vi "Single HWSync LITE.vi"() -> ()   [LabVIEW 2014]
doc: "Use this template to build a producer/consumer design pattern with events to produce queue items. Use this design pattern instead of the User Interface Event Handler pattern for user interfaces when you want to execute code asynchronously in response to an event without slowing the user interface responsiveness."
uses:
  TypeDefs/HAL Config Data.ctl
  APIs/Data Queue/Acquisition Data 1 Sample Cluster.ctl
  APIs/Data Queue/Control Data Cluster.ctl
  APIs/Message Queue/Enqueue Message (Array).vi
  APIs/Message Queue/WINFAS 2 Message Queue.lvlib
  HWSyncLoop/HWSyncLoop.lvlib
  APIs/Data Queue/WINFAS 2 Data Queue.lvlib
panel:
  in  "Config":bool
  in  "LOAD DRIVER":bool
  in  "Disconnect":bool
  in  "Connect":bool
  in  "Sequence:Stop":bool
  in  "Sequence:Start":bool
  in  "Auto-Refresh:Stop":bool
  in  "Auto-Refresh:Start":bool
  in  "Stop Cycle":bool
  in  "Stop Measurement":bool
  in  "Start Measurement":bool
  in  "Start Cycle":bool
  out "TDX":sgl[][](graph)
  out "Valores TDX":sgl[](array[numeric]) format="%0+10.6fmm"
  out "TDX N°":i32[](array[numeric])
  in  "Encoder Zero":bool
  out "DO":bool[][](array[boolean])
  out "DI":bool[][](array[boolean])
  in  "DO Button":bool[][](array[boolean])=[[FALSE, FALSE, FALSE, FALSE, FALSE, FALSE, FALSE, FALSE], [FALSE, FALSE, FALSE, FALSE, FALSE, FALSE, FALSE, FALSE]]
  out "Encoder":sgl(knob) scale=-360.0..360.0 scale format="%.0f°"
  out "Errores":string
  out "Status Bar":string="LOAD"
  out "Driver:":string
  # "Single HWSync LITE"
  # "Entradas Digitales (0-15)"
  # "Salidas Digitales (0-15)"
  # "Salidas Digitales (0-15)"
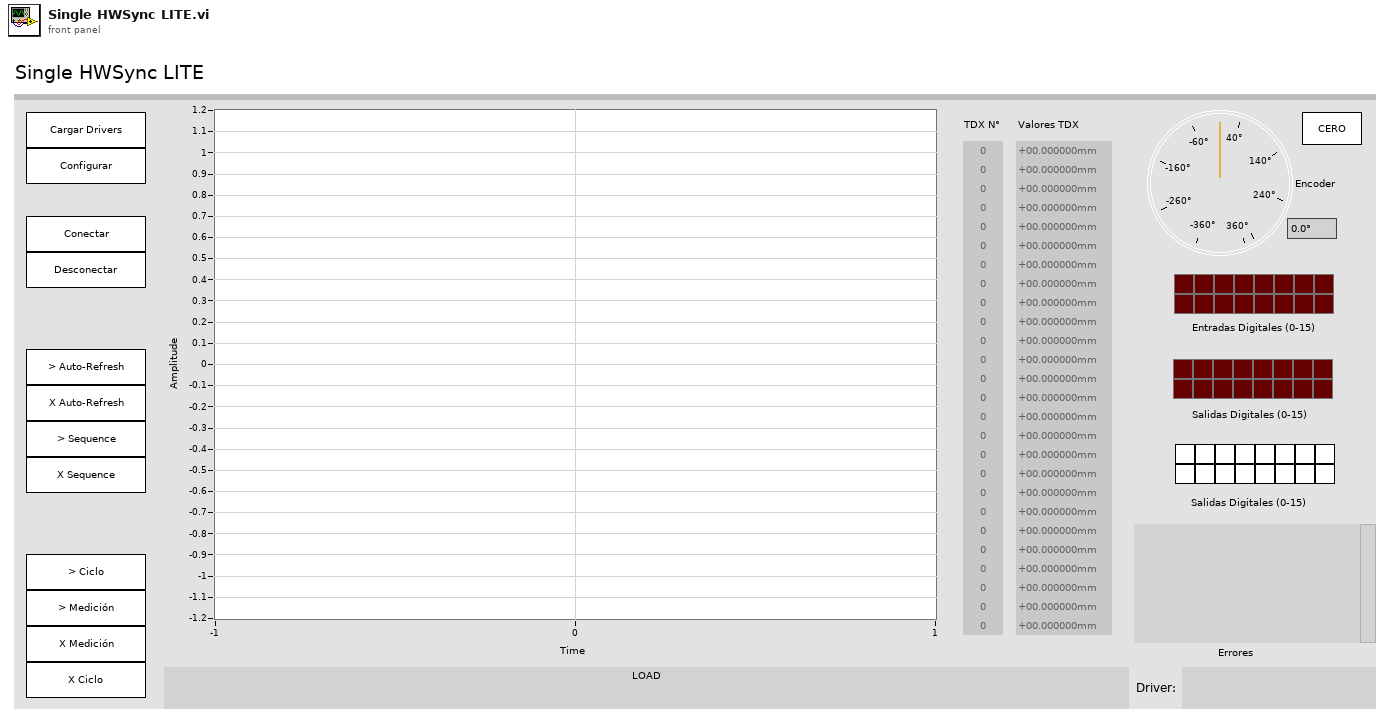
[diagram p1: front panel]
types:
  T1 = typedef "HAL Config Data.ctl" = cluster{"HWSync Index":u32, "Driver Name":string, "Channel Mask":u64}
  T2 = enum32{"invalid app kind", "Development System", "Run Time System", "Student Edition", "Embedded LabVIEW", "Evaluation", "Custom"}
  T3 = typedef "WINFAS 2 Message Queue.lvlib/All Message Queues.ctl" = cluster{"CORE":refnum<queue>, "Event UI":refnum<queue>, "Display UI":refnum<queue>, "MATH":refnum<queue>, "SEQ":refnum<queue>, "DB":refnum<queue>, "ERR":refnum<queue>, "HAL":refnum<queue>, "HWSync1":refnum<queue>, "HWSync2":refnum<queue>, "HWSync3":refnum<queue>, "HWSync4":refnum<queue>, "HWSync5":refnum<queue>, "HWAsync1":refnum<queue>, "HWAsync2":refnum<queue>, "HWAsync3":refnum<queue>, "HWAsync4":refnum<queue>, "HWAsync5":refnum<queue>, "HWAsync6":refnum<queue>, "HWAsync7":refnum<queue>, "HWAsync8":refnum<queue>, "HWAsync9":refnum<queue>, "HWAsync10":refnum<queue>}
  T4 = typedef "WINFAS 2 Data Queue.lvlib/All Data Queues Cluster.ctl" = cluster{"Queues":cluster{"ACQ HWSync1":refnum<queue>, "ACQ HWSync2":refnum<queue>, "ACQ HWSync3":refnum<queue>, "ACQ HWSync4":refnum<queue>, "ACQ HWSync5":refnum<queue>}, "Notifiers":cluster{"Control":cluster{"CTRL HWSync1":refnum<notifier>, "CTRL HWSync2":refnum<notifier>, "CTRL HWSync3":refnum<notifier>, "CTRL HWSync4":refnum<notifier>, "CTRL HWSync5":refnum<notifier>}, "Acquisition":cluster{"ACQ HWSync1":refnum<notifier>, "ACQ HWSync2":refnum<notifier>, "ACQ HWSync3":refnum<notifier>, "ACQ HWSync4":refnum<notifier>, "ACQ HWSync5":refnum<notifier>}, "Async":cluster{"ACQ HWAsync1":refnum<notifier>, "ACQ HWAsync2":refnum<notifier>, "ACQ HWAsync3":refnum<notifier>, "ACQ HWAsync4":refnum<notifier>, "ACQ HWAsync5":refnum<notifier>, "ACQ HWAsync6":refnum<notifier>, "ACQ HWAsync7":refnum<notifier>, "ACQ HWAsync8":refnum<notifier>, "ACQ HWAsync9":refnum<notifier>, "ACQ HWAsync10":refnum<notifier>}}}
  T5 = typedef "WINFAS 2 Data Queue.lvlib/Acquisition Data 1 Sample Cluster.ctl" = cluster{"TDX":sgl[], "Encoder":sgl}
  T6 = typedef "WINFAS 2 Data Queue.lvlib/Control Data Cluster.ctl" = cluster{"Encoder":sgl, "DI":bool[], "DO":bool[]}
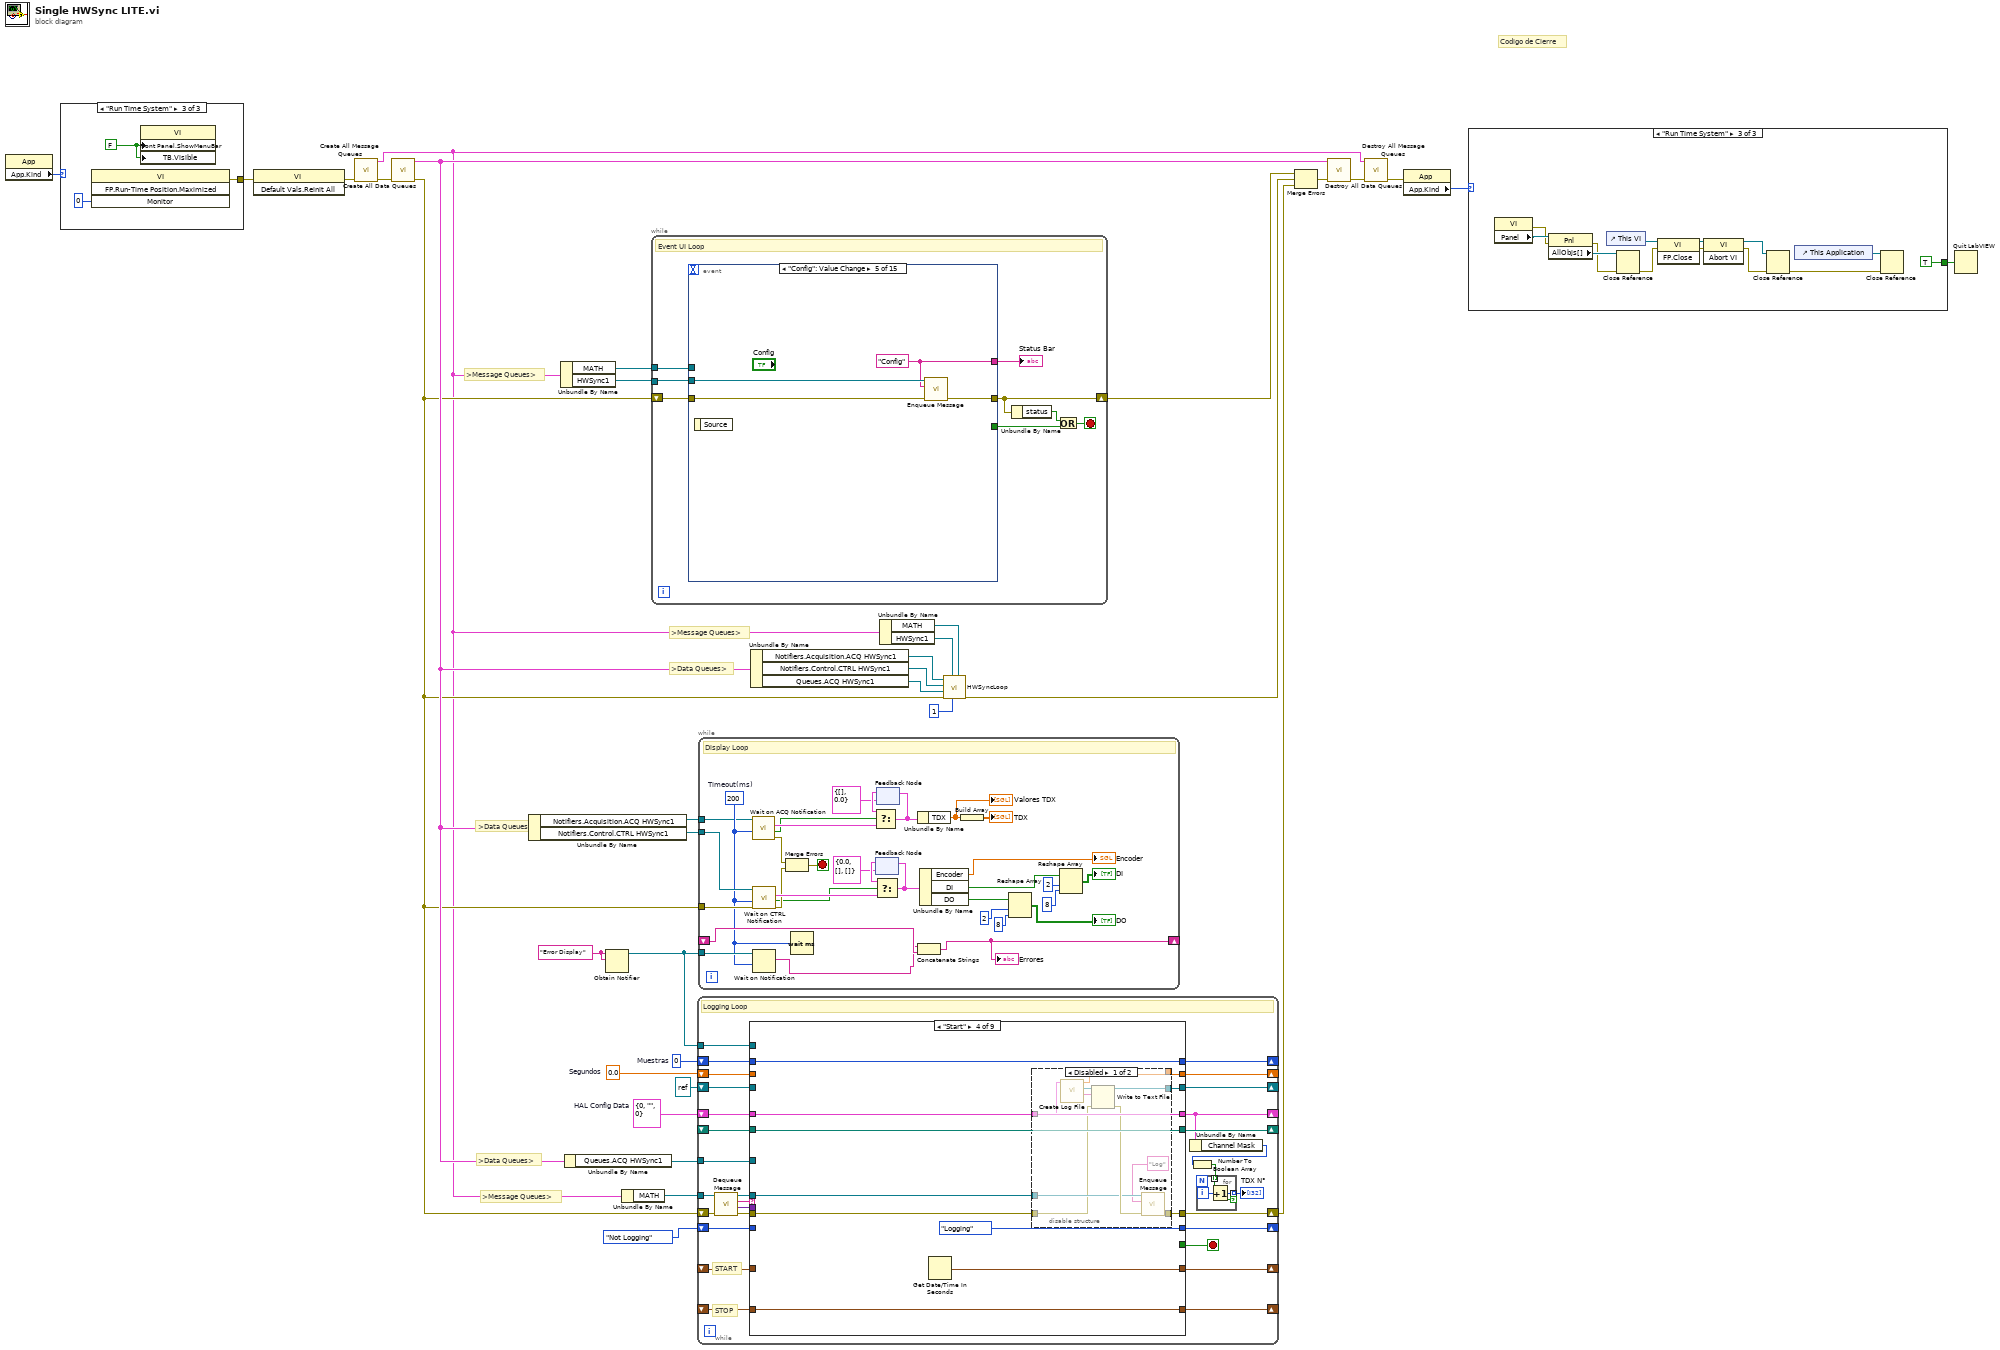
[diagram p0: block diagram]
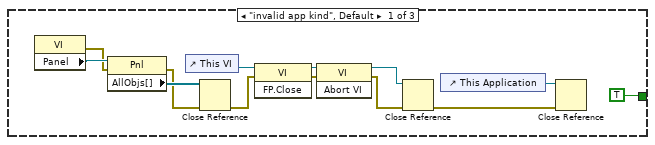
[diagram p4: hidden frame]
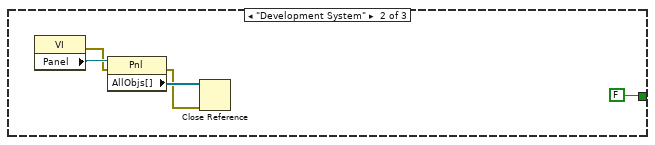
[diagram p5: hidden frame]
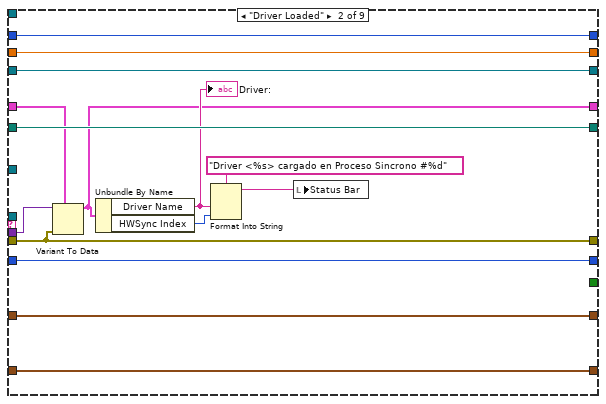
[diagram p7: hidden frame]
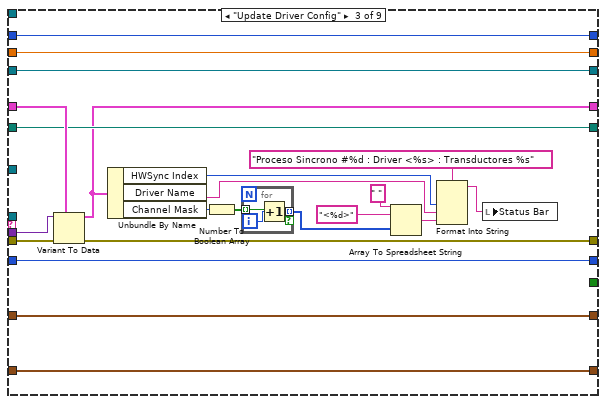
[diagram p8: hidden frame]
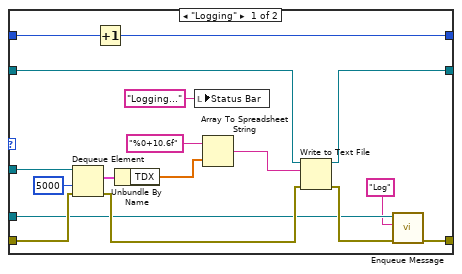
[diagram p11: hidden frame]
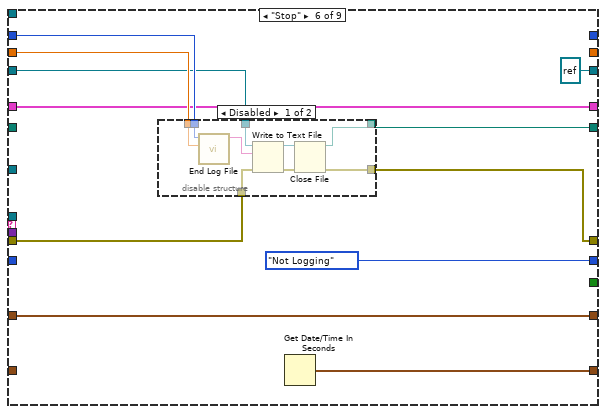
[diagram p12: hidden frame]
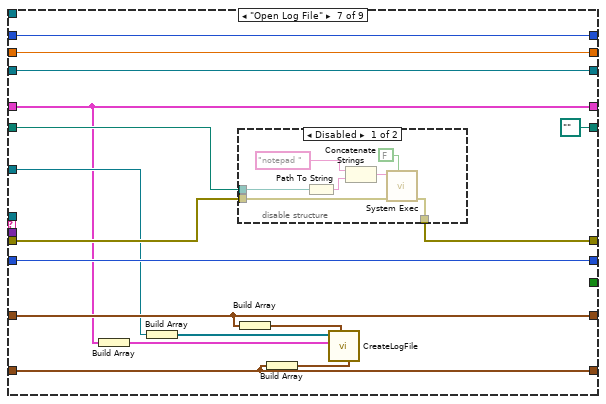
[diagram p14: hidden frame]
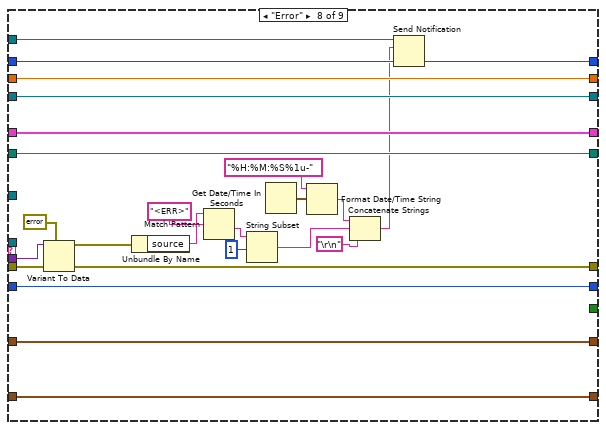
[diagram p16: hidden frame]
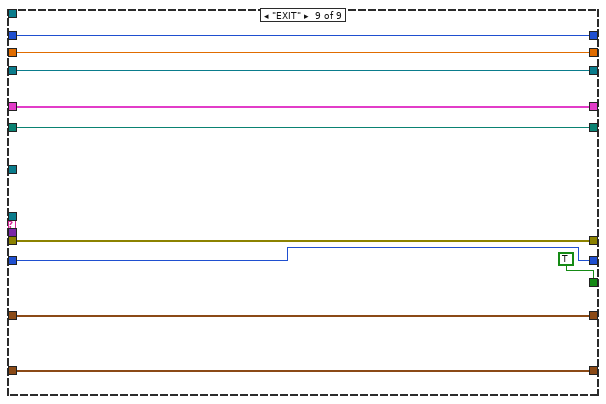
[diagram p17: hidden frame]
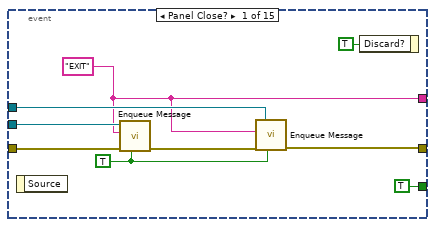
[diagram p18: hidden frame]
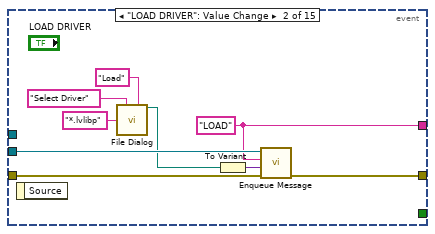
[diagram p19: hidden frame]
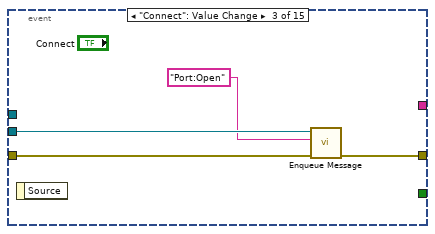
[diagram p20: hidden frame]
diagram:
  w2 = "Error Display" ("name (unnamed)")
  w4 = T1 {"HWSync Index"=0, "Driver Name"="", "Channel Mask"=0}  # HAL Config Data
  w25 = 0.0  # Segundos
  w26 = 0  # Muestras
  # "Codigo de Cierre"
  # ">Message Queues>"
  # ">Data Queues>"
  # ">Message Queues>"
  # ">Data Queues>"
  # ">Data Queues>"
  # ">Message Queues>"
  n1 = property class="App"() -> ("App.Kind"=w21:T2)  [unwired: 2 in, 2 out]
  n2 = case shown="\"Run Time System\"" w21 {
    tunnel: [_ _ w36] -> w20
    frame "invalid app kind", Default {
    }
    frame "Development System" {
    }
    frame "Run Time System" {
      w35 = FALSE ("Front Panel Window:Show Menu Bar")
      n3 = invoke class="VI" method="FP.Run-Time Position.Maximized"("Monitor"=i16 0) -> (error out=w36:errorcluster)  [unwired: 3 in, 3 out]
      n4 = property class="VI"("Front Panel.ShowMenuBar"=w35, "TB.Visible"=w35) -> ()  [unwired: 2 in, 2 out]
    }
  }
  n5 = invoke class="VI" method="Default Vals.Reinit All"(error in=w20) -> (error out=w8:errorcluster)  [unwired: 2 in, 2 out]
  n6 = call "Create All Message Queues.vi"("error in (no error)"=w8) -> ("error out"=w10:errorcluster, "Message Queues Out"=w5:T3)  [unwired: 9 in]
  n7 = call "Create All Data Queues.vi"("Error In"=w10) -> ("Error Out"=w6:errorcluster, "WINFAS 2 Data Queue.lvlib:All Data Queues Cluster"=w9:T4)  [unwired: 9 in]
  n8 = Unbundle By Name(w9) -> ("Notifiers.Acquisition.ACQ HWSync1"=w16:refnum<notifier>, "Notifiers.Control.CTRL HWSync1"=w15:refnum<notifier>)
  n9 = Unbundle By Name(w5) -> ("MATH"=w34:refnum<queue>, "HWSync1"=w30:refnum<queue>)
  n10 = Unbundle By Name(w9) -> ("Queues.ACQ HWSync1"=w14:refnum<queue>)
  n11 = Obtain Notifier(name (unnamed)=w2, notification data type=w2) -> (notifier out=w1:refnum<notifier>)  [unwired: 2 in, 2 out]
  n12 = Unbundle By Name(w5) -> ("MATH"=w27:refnum<queue>)
  n13 = while {
    shift-right: [w42] -> w31
    shift-left: w6 -> [w44]
    tunnel: w34 -> [w45]
    tunnel: w30 -> [w40]
    stop <- w38 stop-if-true
    # "Event UI Loop"
    n14 = event shown="[4] \"Config\": Value Change" {
      selector: _ -> [_ _ _ _ _ _ _ _ _ _ _ _ _ _ _]
      dyn-events: _ -> [_ _ _ _ _ _ _ _ _ _ _ _ _ _ _]
      timeout: _ -> [_ _ _ _ _ _ _ _ _ _ _ _ _ _ _]
      tunnel: w45 -> [w51 _ _ _ _ _ _ w94 w100 _ w111 w121 w130 _ _]
      tunnel: w44 -> [w53 w63 w67 w71 w74 w82 w87 w97 w105 w109 w118 w128 w137 w142 w150]
      tunnel: [w48 w61 w66 w70 w73 w78 w85 w96 w99 _ w112 w122 w131 w138 w149] -> w42
      tunnel: [TRUE ("stop") _ _ _ _ _ _ _ _ _ _ _ _ _ _] -> w43
      tunnel: w40 -> [w54 w62 w65 w69 w75 w81 w86 w95 w103 w108 w117 w127 w136 w140 w152]
      tunnel: [w50 w55 _ _ w72 w77 w84 w89 w101 "Cycle START" ("Message") "Measurement START" ("Message") "Measurement Stop" ("Message") "Cycle Stop" ("Message") _ _] -> w39
      event Panel Close? {
        w52 = TRUE ("Priority Message? (F)")
        w50 = "EXIT" ("String")
        n15 = event-data() -> ()  [unwired: 1 in, 1 out]
        n16 = call-poly "Enqueue Message.vi"("Priority Message? (F)"=w52, "error in (no error)"=w53, "Message"=w50, "Message Queue"=w54) -> ("error out"=w49:errorcluster)  [unwired: 6 in, 1 out]
        n17 = call-poly "Enqueue Message.vi"("Priority Message? (F)"=w52, "error in (no error)"=w49, "Message"=w50, "Message Queue"=w51) -> ("error out"=w48:errorcluster)  [unwired: 6 in, 1 out]
        n18 = event-data("Discard?"=TRUE) -> ()  [unwired: 1 in, 1 out]
      }
      event "LOAD DRIVER": Value Change {
        w55 = "LOAD" ("Message")
        n19 = event-data() -> ()  [unwired: 1 in, 1 out]
        n20 = call "File Dialog"("prompt"="Select Driver", "button label"="Load", "default name"="*.lvlibp") -> ("selected path"=w56:path)  [unwired: 9 in, 3 out]
        n21 = To Variant(anything=w56) -> (Variant=w60:variant)
        n22 = call-poly "Enqueue Message.vi"("error in (no error)"=w63, "Message Data"=w60, "Message"=w55, "Message Queue"=w62) -> ("error out"=w61:errorcluster)  [unwired: 6 in, 1 out]
      }
      event "Connect": Value Change {
        n23 = event-data() -> ()  [unwired: 1 in, 1 out]
        n24 = call-poly "Enqueue Message.vi"("error in (no error)"=w67, "Message"="Port:Open" ("String"), "Message Queue"=w65) -> ("error out"=w66:errorcluster)  [unwired: 7 in, 1 out]
      }
      event "Disconnect": Value Change {
        n25 = event-data() -> ()  [unwired: 1 in, 1 out]
        n26 = call-poly "Enqueue Message.vi"("error in (no error)"=w71, "Message"="Port:Close" ("String"), "Message Queue"=w69) -> ("error out"=w70:errorcluster)  [unwired: 7 in, 1 out]
      }
      event "Config": Value Change {
        w72 = "Config" ("String")
        n27 = event-data() -> ()  [unwired: 1 in, 1 out]
        n28 = call-poly "Enqueue Message.vi"("error in (no error)"=w74, "Message"=w72, "Message Queue"=w75) -> ("error out"=w73:errorcluster)  [unwired: 7 in, 1 out]
      }
      event "Auto-Refresh:Start": Value Change {
        w77 = "Auto-Refresh:Start" ("Message")
        n29 = event-data() -> ()  [unwired: 1 in, 1 out]
        n30 = call-poly "Enqueue Message.vi"("error in (no error)"=w82, "Message"="Auto-Refresh:Init" ("String"), "Message Queue"=w81) -> ("error out"=w79:errorcluster, "dup Message Queue"=w76:refnum<queue>)  [unwired: 7 in]
        n31 = call-poly "Enqueue Message.vi"("error in (no error)"=w79, "Message"=w77, "Message Queue"=w76) -> ("error out"=w78:errorcluster)  [unwired: 7 in, 1 out]
      }
      event "Auto-Refresh:Stop": Value Change {
        w84 = "Auto-Refresh:Stop" ("Message")
        n32 = event-data() -> ()  [unwired: 1 in, 1 out]
        n33 = call-poly "Enqueue Message.vi"("Priority Message? (F)"=TRUE, "error in (no error)"=w87, "Message"=w84, "Message Queue"=w86) -> ("error out"=w85:errorcluster)  [unwired: 6 in, 1 out]
      }
      event "Sequence:Start": Value Change {
        w89 = "Sequence:Start" ("Message")
        n34 = event-data() -> ()  [unwired: 1 in, 1 out]
        n35 = call-poly "Enqueue Message.vi"("error in (no error)"=w97, "Message"="Sequence:Init" ("String"), "Message Queue"=w95) -> ("error out"=w92:errorcluster, "dup Message Queue"=w88:refnum<queue>)  [unwired: 7 in]
        n36 = call-poly "Enqueue Message.vi"("error in (no error)"=w92, "Message"=w89, "Message Queue"=w88) -> ("error out"=w91:errorcluster)  [unwired: 7 in, 1 out]
        n37 = call-poly "Enqueue Message.vi"("error in (no error)"=w91, "Message"="Start", "Message Queue"=w94) -> ("error out"=w96:errorcluster)  [unwired: 7 in, 1 out]
      }
      event "Sequence:Stop": Value Change {
        w101 = "Sequence:Stop" ("Message")
        n38 = event-data() -> ()  [unwired: 1 in, 1 out]
        n39 = call-poly "Enqueue Message.vi"("Priority Message? (F)"=TRUE, "error in (no error)"=w105, "Message"=w101, "Message Queue"=w103) -> ("error out"=w104:errorcluster)  [unwired: 6 in, 1 out]
        n40 = call-poly "Enqueue Message.vi"("error in (no error)"=w104, "Message Array"=string[] ["Stop", "Open Log File"], "Message Queue"=w100) -> ("error out"=w99:errorcluster)  [unwired: 7 in, 1 out]
      }
      event "Start Cycle": Value Change {
        n41 = event-data() -> ()  [unwired: 1 in, 2 out]
        n42 = call-poly "Enqueue Message.vi"("error in (no error)"=w109, "Message Array"=string[] ["Auto-Refresh:Init", "Auto-Refresh:Start", "Diagnostic:Cycle"], "Message Queue"=w108) -> ()  [unwired: 7 in, 2 out]
      }
      event "Start Measurement": Value Change {
        n43 = event-data() -> ()  [unwired: 1 in, 6 out]
        n44 = call-poly "Enqueue Message.vi"("Priority Message? Array"=bool[] [TRUE, FALSE, FALSE, FALSE], "error in (no error)"=w118, "Message Array"=string[] ["Auto-Refresh:Stop", "Sequence:Init", "Sequence:Start", "Diagnostic:Measurement"], "Message Queue"=w117) -> ("error out"=w113:errorcluster)  [unwired: 6 in, 1 out]
        n45 = call-poly "Enqueue Message.vi"("error in (no error)"=w113, "Message"="Start", "Message Queue"=w111) -> ("error out"=w112:errorcluster)  [unwired: 7 in, 1 out]
      }
      event "Stop Measurement": Value Change {
        n46 = event-data() -> ()  [unwired: 1 in, 6 out]
        n47 = call-poly "Enqueue Message.vi"("Priority Message? Array"=bool[] [TRUE, FALSE, FALSE], "error in (no error)"=w128, "Message Array"=string[] ["Sequence:Stop", "Auto-Refresh:Init", "Auto-Refresh:Start"], "Message Queue"=w127) -> ("error out"=w123:errorcluster)  [unwired: 6 in, 1 out]
        n48 = call-poly "Enqueue Message.vi"("Priority Message? (F)"=TRUE, "error in (no error)"=w123, "Message"="Stop", "Message Queue"=w121) -> ("error out"=w122:errorcluster)  [unwired: 6 in, 1 out]
      }
      event "Stop Cycle": Value Change {
        n49 = event-data() -> ()  [unwired: 1 in, 6 out]
        n50 = call-poly "Enqueue Message.vi"("Priority Message? Array"=bool[] [TRUE], "error in (no error)"=w137, "Message Array"=string[] ["Auto-Refresh:Stop"], "Message Queue"=w136) -> ("error out"=w132:errorcluster)  [unwired: 6 in, 1 out]
        n51 = call-poly "Enqueue Message.vi"("error in (no error)"=w132, "Message"="Open Log File", "Message Queue"=w130) -> ("error out"=w131:errorcluster)  [unwired: 7 in, 1 out]
      }
      event "Encoder Zero": Value Change {
        n52 = event-data() -> ()  [unwired: 1 in, 6 out]
        n53 = call-poly "Enqueue Message.vi"("Priority Message? (F)"=TRUE, "error in (no error)"=w142, "Message"="Encoder Zero", "Message Queue"=w140) -> ("error out"=w138:errorcluster)  [unwired: 6 in, 1 out]
      }
      event "DO Button": Value Change {
        n54 = event-data() -> ()  [unwired: 1 in, 1 out]
        n55 = Reshape Array("DO Button", 16 ("dimension size")) -> (w143:bool[])
        n56 = Boolean Array To Number(Boolean array=w143) -> (number=w146:u32)
        n57 = To Variant(anything=w146) -> (Variant=w147:variant)
        n58 = call "Enqueue Message (Single).vi"("Priority Message? (F)"=TRUE, "error in (no error)"=w150, "Message Data"=w147, "Message"="Digital Out Write", "Message Queue"=w152) -> ("error out"=w149:errorcluster)  [unwired: 5 in, 1 out]
      }
    }
    "Status Bar" <- w39
    n59 = Unbundle By Name(w42) -> ("status"=w41:bool)
    n60 = Or(x=w41, y=w43) -> (x .or. y?=w38:bool)
  }
  n61 = while {
    tunnel: w14 -> [w178]
    tunnel: w27 -> [w177]
    shift-right: [w180] -> _
    shift-left: refnum<file> refnum ("refnum out") -> [w179]
    shift-right: [w174] -> w7
    shift-left: w6 -> [w173]
    shift-right: [w172] -> _
    shift-left: w25 -> [w171]
    shift-right: [w170] -> _
    shift-left: w26 -> [w169]
    shift-right: [w160] -> _
    shift-left: w4 -> [w167]
    shift-right: [w165] -> _
    shift-left: _ -> [w164]
    shift-right: [w162] -> _
    shift-left: enum16{"Logging", "Not Logging"}."Not Logging" -> [w163]
    tunnel: w1 -> [w161]
    shift-right: [w156] -> _
    shift-left: _ -> [w155]
    shift-right: [w154] -> _
    shift-left: _ -> [w153]
    stop <- w176 stop-if-true
    # "STOP"
    # "START"
    # "Logging Loop"
    n62 = call "Dequeue Message.vi"("error in (no error)"=w173, "Message Queue"=w177) -> ("error out"=w175:errorcluster, "Message Data"=w166:variant, "Message"=w181:string, "dup Message Queue"=w168:refnum<queue>)  [unwired: 6 in]
    n63 = case shown="\"Start\"" w181 {
      tunnel: [w193 w208 w230 w244 w266 refnum<file> refnum ("refnum out") w324 w350 w365] -> w180
      tunnel: w179 -> [w193 w208 w230 _ w267 w296 w324 w350 w365]
      tunnel: w178 -> [_ _ _ _ w268 _ w312 _ _]
      tunnel: w168 -> [_ _ _ w243 w263 _ _ _ _]
      tunnel: [_ _ _ _ _ _ _ _ TRUE] -> w176
      tunnel: w175 -> [w192 w203 w227 w239 w265 w292 w321 w348 w363]
      tunnel: [w192 w203 w226 w242 w264 w293 w320 w346 w363] -> w174
      tunnel: [w190 w207 w229 w241 w262 _ w323 w355 w361] -> w172
      tunnel: w171 -> [w190 w207 w229 _ w262 w298 w323 w355 w361]
      tunnel: [w191 w206 w228 w240 w260 _ w322 w354 w362] -> w170
      tunnel: w169 -> [w191 w206 w228 w240 w261 w297 w322 w354 w362]
      tunnel: w167 -> [w189 w197 w225 w238 w259 w295 w310 w352 w360]
      tunnel: [w189 w196 w221 w238 w259 w295 w310 w352 w360] -> w160
      tunnel: w166 -> [_ w202 w224 _ _ _ _ w349 _]
      tunnel: [w188 w205 w223 w237 w258 w294 path "" ("path") w353 w359] -> w165
      tunnel: w164 -> [w188 w205 w223 w237 w258 _ w319 w353 w359]
      tunnel: w163 -> [w187 w204 w222 _ w257 _ w317 w351 w358]
      tunnel: [w187 w204 w222 enum16{"Logging", "Not Logging"}."Logging" w257 enum16{"Logging", "Not Logging"}."Not Logging" w317 w351 w358] -> w162
      tunnel: w161 -> [_ _ _ _ _ _ _ w335 _]
      tunnel: [w186 w195 w210 w235 w256 w290 w316 w333 w357] -> w156
      tunnel: w155 -> [w186 w195 w210 _ w256 w290 w316 w333 w357]
      tunnel: [w185 w194 w209 w234 w255 w289 w315 w332 w356] -> w154
      tunnel: w153 -> [w185 w194 w209 w234 w255 _ w315 w332 w356]
      frame Default {
      }
      frame "Driver Loaded" {
        n64 = Variant To Data(error in=w203, type=w197, Variant=w202) -> (data=w196:T1)  [unwired: 1 out]
        n65 = Unbundle By Name(w196) -> ("Driver Name"=w198:string, "HWSync Index"=w199:u32)
        "Driver:" <- w198
        n66 = Format Into String(format string="Driver <%s> cargado en Proceso Sincrono #%d", w198, w199) -> (resulting string=w200:string)  [unwired: 2 in, 1 out]
        n67 = local write "Status Bar"(w200) -> ()
      }
      frame "Update Driver Config" {
        n68 = Variant To Data(error in=w227, type=w225, Variant=w224) -> (data=w221:T1, error out=w226:errorcluster)
        n69 = Unbundle By Name(w221) -> ("HWSync Index"=w219:u32, "Driver Name"=w218:string, "Channel Mask"=w216:u64)
        n70 = Number To Boolean Array(number=w216) -> (Boolean array=w215:bool[])
        n71 = for {
          tunnel: w215 -> [w231] mode=indexing
          tunnel: [w232] -> w214 mode=indexing if=w231
          i -> [w233]
          n72 = Increment(x=w233) -> (x+1=w232:i32)
        }
        n73 = Array To Spreadsheet String(delimiter (Tab)=" ", array=w214, 3:"<%d>" ("format string")) -> (spreadsheet string=w212:string)
        n74 = Format Into String(format string="Proceso Sincrono #%d : Driver <%s> : Transductores %s", w219, w218, w212) -> (resulting string=w217:string)  [unwired: 2 in, 1 out]
        n75 = local write "Status Bar"(w217) -> ()
      }
      frame "Start" {
        n76 = Get Date/Time In Seconds() -> (seconds since 1Jan1904=w235:timestamp)
        n77 = disable-structure shown="Disabled" {
          disable-tunnel: [w254 _] -> w244
          disable-tunnel: w243 -> [w252 _]
          disable-tunnel: [w250 _] -> w242
          disable-tunnel: [w249 _] -> w241
          disable-tunnel: w239 -> [w246 _]
          disable-tunnel: w238 -> [w245 _]
          frame Disabled {
            n78 = call "Create Log File.vi"("HAL Config Data"=w245) -> ("String"=w247:string, "Byte Stream File out"=w248:refnum<file>, "Seconds"=w249:dbl)  [unwired: 8 in]
            n79 = Write to Text File(file (use dialog)=w248, text=w247, error in=w246) -> (refnum out=w254:refnum<file>, error out=w253:errorcluster)  [unwired: 1 in, 1 out]
            n80 = call-poly "Enqueue Message.vi"("error in (no error)"=w253, "Message"="Log", "Message Queue"=w252) -> ("error out"=w250:errorcluster)  [unwired: 7 in, 1 out]
          }
          frame Enabled {
          }
        }
      }
      frame "Log" {
        n81 = case shown="\"Not Logging\", Default" w257 {
          tunnel: w268 -> [w285 _]
          tunnel: w267 -> [w283 w287]
          tunnel: [w282 w287] -> w266
          tunnel: w265 -> [w281 w286]
          tunnel: [w277 w286] -> w264
          tunnel: w263 -> [w276 _]
          tunnel: w261 -> [w274 w288]
          tunnel: [w272 w288] -> w260
          frame "Logging" {
            n82 = Dequeue Element(queue=w285, timeout in ms (-1)=5000, error in (no error)=w281) -> (element=w284:T5, error out=w280:errorcluster)  [unwired: 2 out]
            n83 = Increment(x=w274) -> (x+1=w272:i32)
            n84 = Unbundle By Name(w284) -> ("TDX"=w271:sgl[])
            n85 = local write "Status Bar"("Logging..." ("Status Bar")) -> ()
            n86 = Array To Spreadsheet String(array=w271, 3:"%0+10.6f" ("format string")) -> (spreadsheet string=w269:string)  [unwired: 1 in]
            n87 = Write to Text File(file (use dialog)=w283, text=w269, error in=w280) -> (refnum out=w282:refnum<file>, error out=w278:errorcluster)  [unwired: 1 in, 1 out]
            n88 = call-poly "Enqueue Message.vi"("error in (no error)"=w278, "Message"="Log", "Message Queue"=w276) -> ("error out"=w277:errorcluster)  [unwired: 7 in, 1 out]
          }
          frame "Not Logging", Default {
          }
        }
      }
      frame "Stop" {
        n89 = disable-structure shown="Disabled" {
          disable-tunnel: w298 -> [w307 _]
          disable-tunnel: w297 -> [w306 _]
          disable-tunnel: w296 -> [w304 _]
          disable-tunnel: [w302 _] -> w294
          disable-tunnel: [w301 _] -> w293
          disable-tunnel: w292 -> [w300 _]
          frame Disabled {
            n90 = call "End Log File.vi"("Seconds"=w307, "Muestras totales"=w306) -> ("String"=w305:string)  [unwired: 9 in]
            n91 = Write to Text File(file (use dialog)=w304, text=w305, error in=w300) -> (refnum out=w308:refnum<file>, error out=w303:errorcluster)  [unwired: 1 in, 1 out]
            n92 = Close File(refnum=w308, error in=w303) -> (path=w302:path, error out=w301:errorcluster)
          }
          frame Enabled {
          }
        }
        n93 = Get Date/Time In Seconds() -> (seconds since 1Jan1904=w289:timestamp)
      }
      frame "Open Log File" {
        n94 = Build Array(w310) -> (w309:T1[])
        n95 = Build Array(w312) -> (w311:refnum<queue>[])
        n96 = disable-structure shown="Disabled" {
          disable-tunnel: w321 -> [w327 _]
          disable-tunnel: [w326 _] -> w320
          disable-tunnel: w319 -> [w325 _]
          frame Disabled {
            n97 = Path To String(path=w325) -> (string=w330:string)
            n98 = Concatenate Strings("notepad ", w330) -> (w328:string)
            n99 = call <vilib>:"System Exec.vi"("wait until completion? (T)"=FALSE, "error in (no error)"=w327, "command line"=w328) -> ("error out"=w326:errorcluster)  [unwired: 5 in, 3 out]
          }
          frame Enabled {
          }
        }
        n100 = Build Array(w316) -> (w314:timestamp[])
        n101 = Build Array(w315) -> (w313:timestamp[])
        n102 = call "CreateLogFile.vi"("Stop Time"=w313, "Start Time"=w314, "HAL Config"=w309, "ACQ Queues"=w311) -> ()  [unwired: 8 in]
      }
      frame "Error" {
        n103 = Variant To Data(error in=w348, type=errorcluster {"status"=FALSE, "code"=0, "source"=""} ("error out"), Variant=w349) -> (data=w345:errorcluster, error out=w346:errorcluster)
        n104 = Unbundle By Name(w345) -> ("source"=w343:string)
        n105 = Match Pattern(string=w343, regular expression="<ERR>") -> (after substring=w338:string)  [unwired: 1 in, 3 out]
        n106 = String Subset(string=w338, offset (0)=1) -> (substring=w337:string)  [unwired: 1 in]
        n107 = Get Date/Time In Seconds() -> (seconds since 1Jan1904=w342:timestamp)
        n108 = Format Date/Time String(time format string (%c)="%H:%M:%S%1u-", seconds (now)=w342) -> (date/time string=w339:string)  [unwired: 1 in]
        n109 = Concatenate Strings(w339, w337, "\r\n") -> (w334:string)
        n110 = Send Notification(notification=w334, notifier=w335) -> ()  [unwired: 1 in, 2 out]
      }
      frame "EXIT" {
      }
    }
    n111 = Unbundle By Name(w160) -> ("Channel Mask"=w159:u64)
    n112 = Number To Boolean Array(number=w159) -> (Boolean array=w158:bool[])
    n113 = for {
      tunnel: w158 -> [w182] mode=indexing
      tunnel: [w183] -> w157 mode=indexing if=w182
      i -> [w184]
      n114 = Increment(x=w184) -> (x+1=w183:i32)
    }
    "TDX N°" <- w157
  }
  n115 = while {
    tunnel: w16 -> [w368]
    tunnel: w15 -> [w392]
    tunnel: w6 -> [w384]
    tunnel: w1 -> [w374]
    shift-right: [w372] -> _
    shift-left: _ -> [w373]
    stop <- w385 stop-if-true
    w369 = 200  # Timeout(ms)
    # "Display Loop"
    n116 = call "Wait on ACQ Notification.vi"("timeout in ms (-1)"=w369, "ACQ Data Notifier in"=w368) -> ("error out"=w380:errorcluster, "timed out?"=w367:bool, "1 Sample"=w388:T5)  [unwired: 6 in, 1 out]
    n117 = call "Wait on CTRL Notification.vi"("error in (no error)"=w384, "timeout in ms (-1)"=w369, "CTRL Data Notifier in"=w392) -> ("error out"=w381:errorcluster, "timed out?"=w366:bool, "Control Data"=w391:T6)  [unwired: 5 in, 1 out]
    n118 = Wait on Notification(notifier=w374, timeout in ms (-1)=w369) -> (notification=w370:string)  [unwired: 2 in, 3 out]
    n119 = Merge Errors(w380, w381) -> (w385:errorcluster)
    n120 = Wait (ms)(milliseconds to wait=w369) -> ()  [unwired: 1 out]
    n121 = feedback #1(T6 {"Encoder"=0.0, "DI"=[], "DO"=[]} ("Control Data")) -> (w390:T6)
    n122 = Select(t=w390, s=w366, f=w391) -> (s? t:f=w389:T6)
    n123 = feedback-in #1(w389) -> ()
    n124 = feedback #2(T5 {"TDX"=[], "Encoder"=0.0} ("1 Sample")) -> (w387:T5)
    n125 = Select(t=w387, s=w367, f=w388) -> (s? t:f=w386:T5)
    n126 = feedback-in #2(w386) -> ()
    n127 = Unbundle By Name(w386) -> ("TDX"=w371:sgl[])
    "Valores TDX" <- w371
    n128 = Concatenate Strings(w370, w373) -> (w372:string)
    "Errores" <- w372
    n129 = Unbundle By Name(w389) -> ("Encoder"=→"Encoder":sgl, "DI"=w397:bool[], "DO"=w394:bool[])
    n130 = Build Array(w371) -> (→"TDX":sgl[][])
    n131 = Reshape Array(w394, 2 ("index"), 8 ("dimension size")) -> (→"DO":bool[][])
    n132 = Reshape Array(w397, 2 ("index"), 8 ("dimension size")) -> (→"DI":bool[][])
  }
  n133 = Unbundle By Name(w9) -> ("Notifiers.Acquisition.ACQ HWSync1"=w19:refnum<notifier>, "Notifiers.Control.CTRL HWSync1"=w18:refnum<notifier>, "Queues.ACQ HWSync1"=w17:refnum<queue>)
  n134 = Unbundle By Name(w5) -> ("MATH"=w33:refnum<queue>, "HWSync1"=w32:refnum<queue>)
  n135 = call "HWSyncLoop.vi"("HAL"=w33, "Index"=u32 1 ("Num of Loop"), "HWSync"=w32, "error in"=w6, "ACQ Data Queue"=w17, "CTRL Data Notifier"=w18, "ACQ Data Notifier"=w19) -> ("error out"=w29:errorcluster)  [unwired: 4 in]
  n136 = Merge Errors(w31, w29, w7) -> (w13:errorcluster)
  n137 = call "Destroy All Data Queues.vi"("Error In"=w13, "WINFAS 2 Data Queue.lvlib:All Data Queues Cluster"=w9) -> ("Error Out"=w12:errorcluster)  [unwired: 9 in]
  n138 = call "Destroy All Message Queues.vi"("error in (no error)"=w12, "Message Queues Out"=w5) -> ("error out"=w11:errorcluster)  [unwired: 9 in]
  n139 = property class="App"(error in=w11) -> ("App.Kind"=w23:T2)  [unwired: 1 in, 2 out]
  n140 = case shown="\"Run Time System\"" w23 {
    tunnel: [TRUE FALSE TRUE] -> w22
    frame "invalid app kind", Default {
      n141 = property class="VI"() -> (error out=w398:errorcluster, "Panel"=w408:refnum<vi>)  [unwired: 2 in, 1 out]
      n142 = property class="Pnl"(reference=w408, error in=w398) -> (error out=w399:errorcluster, "AllObjs[]"=w407:refnum<vi>[])  [unwired: 1 out]
      n143 = control-ref of="This VI"() -> (w405:refnum<vi>)
      n144 = Close Reference(reference=w407, error in (no error)=w399) -> (error out=w404:errorcluster)
      n145 = invoke class="VI" method="FP.Close"(reference=w405, error in=w404) -> (reference out=w403:refnum<vi>, error out=w402:errorcluster)  [unwired: 1 in, 1 out]
      n146 = invoke class="VI" method="Abort VI"(reference=w403, error in=w402) -> (reference out=w400:refnum<vi>, error out=w401:errorcluster)  [unwired: 1 in, 1 out]
      n147 = Close Reference(reference=w400, error in (no error)=w401) -> (error out=w409:errorcluster)
      n148 = control-ref of="This Application"() -> (w410:refnum<vi>)
      n149 = Close Reference(reference=w410, error in (no error)=w409) -> ()  [unwired: 1 out]
    }
    frame "Development System" {
      n150 = property class="VI"() -> (error out=w411:errorcluster, "Panel"=w415:refnum<vi>)  [unwired: 2 in, 1 out]
      n151 = property class="Pnl"(reference=w415, error in=w411) -> (error out=w412:errorcluster, "AllObjs[]"=w414:refnum<vi>[])  [unwired: 1 out]
      n152 = Close Reference(reference=w414, error in (no error)=w412) -> ()  [unwired: 1 out]
    }
    frame "Run Time System" {
      n153 = property class="VI"() -> (error out=w416:errorcluster, "Panel"=w426:refnum<vi>)  [unwired: 2 in, 1 out]
      n154 = property class="Pnl"(reference=w426, error in=w416) -> (error out=w417:errorcluster, "AllObjs[]"=w425:refnum<vi>[])  [unwired: 1 out]
      n155 = control-ref of="This VI"() -> (w423:refnum<vi>)
      n156 = Close Reference(reference=w425, error in (no error)=w417) -> (error out=w422:errorcluster)
      n157 = invoke class="VI" method="FP.Close"(reference=w423, error in=w422) -> (reference out=w421:refnum<vi>, error out=w420:errorcluster)  [unwired: 1 in, 1 out]
      n158 = invoke class="VI" method="Abort VI"(reference=w421, error in=w420) -> (reference out=w418:refnum<vi>, error out=w419:errorcluster)  [unwired: 1 in, 1 out]
      n159 = Close Reference(reference=w418, error in (no error)=w419) -> (error out=w427:errorcluster)
      n160 = control-ref of="This Application"() -> (w428:refnum<vi>)
      n161 = Close Reference(reference=w428, error in (no error)=w427) -> ()  [unwired: 1 out]
    }
  }
  n162 = Quit LabVIEW(quit? (T)=w22) -> ()
